vi "sort.volume.issues.vi"(8 "error in":errorcluster, 10 "issues path":path=path "D:/Comics/data/cv_issues", 11 "volume path":path) -> (0 "error out":errorcluster)   [LabVIEW 2024]
uses:
  definitions/local_issue.ctl
  definitions/comicvine_issue.generic_credit.ctl
  definitions/comicvine_issue.associated_image.ctl
  definitions/comicvine_issue.person_credit.ctl
  <vilib>/addons/_JKI.lib/Serialization/JSON/JKI JSON Serialization.lvlib
panel:
  out "sorted array":T1(array[cluster])
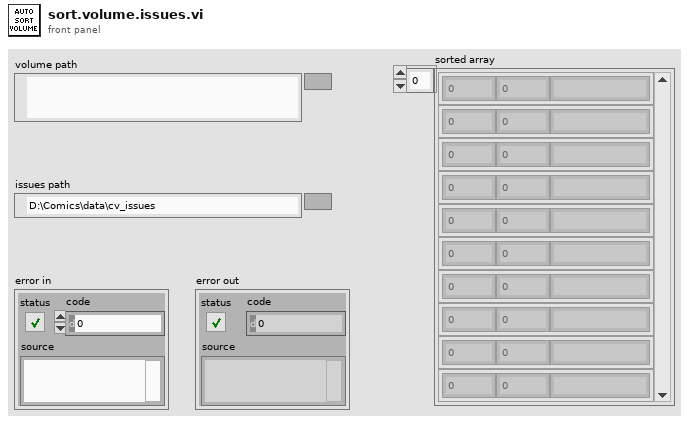
[diagram p1: front panel]
types:
  T1 = cluster{dbl, "issue_id":i32, "issue_number":string}[]
  T2 = typedef "local_volume.ctl" = cluster{"id":i32, "name":string, "sortable_name":string, "aliases":string[], "description":string, "site_detail_url":string, "count_of_issues":i32, "start_year":i32, "publisher_id":i32, "issue_ids":i32[], "date_last_updated":timestamp, "volume":i32, "cv_id":string, "volume type":T3}
  T3 = typedef "volume.type--enum.ctl" = enum16{"Ongoing", "Limited Series", "Annual", "One Shot", "Reprint/Document"}
  T4 = typedef "local_issue.ctl" = cluster{"cover_date":timestamp, "id":i32, "cv_id":string, "name":string, "sortable_name":string, "issue_number":string, "deck":string, "description":string, "volume":T5, "store_date":timestamp, "date_last_updated":timestamp, "site_detail_url":string, "cover_url":string, "associated_images":T6[], "characters":T5[], "concepts":T5[], "creators":T7[], "storyArcs":T5[], "teams":T5[]}
  T5 = typedef "comicvine_issue.generic_credit.ctl" = cluster{"id":i32, "name":string}
  T6 = typedef "comicvine_issue.associated_image.ctl" = cluster{"original_url":string, "id":i32}
  T7 = typedef "comicvine_issue.person_credit.ctl" = cluster{"id":i32, "name":string, "role":string}
  T8 = cluster{dbl, "issue_id":i32, "issue_number":string}
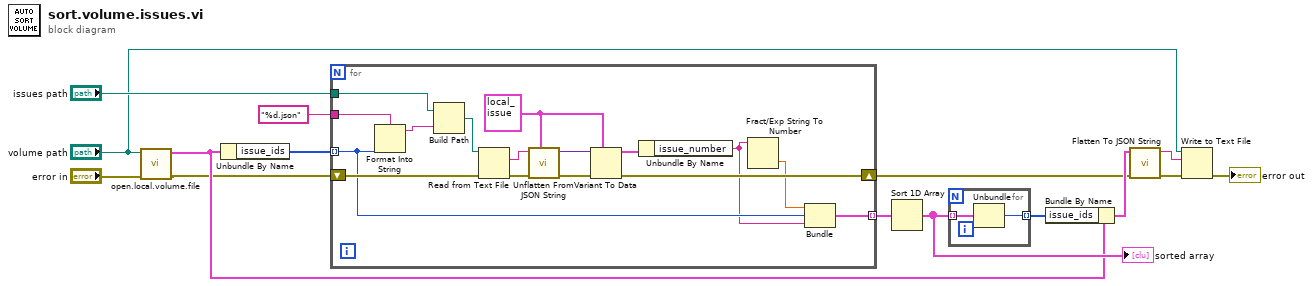
[diagram p0: block diagram]
diagram:
  n1 = call "open.local.volume.file.vi"("error in (no error)"="error in", "volume json"="volume path") -> ("error out"=w1:errorcluster, "volume"=w3:T2)  [unwired: 8 in]
  n2 = Unbundle By Name(w3) -> ("issue_ids"=w15:i32[])
  n3 = for {
    tunnel: w15 -> [w18] mode=indexing
    tunnel: "%d.json" -> [w31]
    tunnel: "issues path" -> [w29]
    shift-right: [w25] -> w9
    shift-left: w1 -> [w26]
    tunnel: [w17] -> w12 mode=indexing
    w21 = T4 {"cover_date"=timestamp(0 s since 1904-01-01), "id"=0, "cv_id"="", "name"="", "sortable_name"="", "issue_number"="", "deck"="", "description"="", "volume"={"id"=0, "name"=""}, "store_date"=timestamp(0 s since 1904-01-01), "date_last_updated"=timestamp(0 s since 1904-01-01), "site_detail_url"="", "cover_url"="", "associated_images"=[], "characters"=[], "concepts"=[], "creators"=[], "storyArcs"=[], "teams"=[]} ("issue")
    n4 = Format Into String(format string=w31, w18) -> (resulting string=w30:string)  [unwired: 2 in, 1 out]
    n5 = Build Path(base path=w29, name or relative path=w30) -> (appended path=w24:path)
    n6 = Read from Text File(file (use dialog)=w24, error in=w26) -> (text=w23:string, error out=w27:errorcluster)  [unwired: 2 in, 2 out]
    n7 = call <vilib>:"Unflatten From JSON String.vi"("Type and Defaults"=w21, "error in (no error)"=w27, "JSON String"=w23) -> ("error out"=w28:errorcluster, "Variant"=w22:variant)  [unwired: 7 in]
    n8 = Variant To Data(error in=w28, type=w21, Variant=w22) -> (data=w20:T4, error out=w25:errorcluster)
    n9 = Unbundle By Name(w20) -> ("issue_number"=w16:string)
    n10 = Fract/Exp String To Number(string=w16) -> (number=w19:dbl)  [unwired: 3 in, 1 out]
    n11 = Bundle(w19, "issue_id"=w18, "issue_number"=w16) -> (w17:T8)  [unwired: 1 in]
  }
  n12 = Sort 1D Array(array=w12) -> (sorted array=w5:T1)
  "sorted array" <- w5
  n13 = for {
    tunnel: w5 -> [w33] mode=indexing
    tunnel: [w32] -> w11 mode=indexing
    n14 = Unbundle(w33) -> ("issue_id"=w32:i32)  [unwired: 2 out]
  }
  n15 = Bundle By Name(cluster=w3, "issue_ids"=w11) -> (w10:T2)
  n16 = call <vilib>:"Flatten To JSON String.vi"("error in (no error)"=w9, "Variant"=w10) -> ("error out"=w8:errorcluster, "JSON String"=w7:string)  [unwired: 8 in]
  n17 = Write to Text File(file (use dialog)="volume path", text=w7, error in=w8) -> (error out=→"error out":errorcluster)  [unwired: 1 in, 2 out]
